vi "dfd_Adjust Height.vi"(9 "origin":cluster{"left":i16, "top":i16}, 10 "fraction rect":T1) -> (2 "rect out":T1)   [LabVIEW 2017, in "NI_DigFilter_Process.lvlib"]
uses:
  <vilib>/addons/Digital Filter Design/NI_DigFilter_Process.lvlib
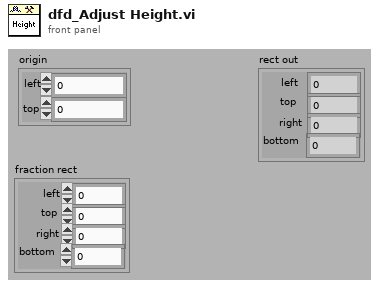
[diagram p1: front panel]
types:
  T1 = cluster{"left":i16, "top":i16, "right":i16, "bottom":i16}
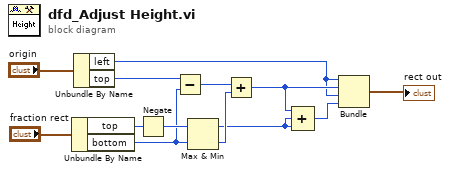
[diagram p0: block diagram]
diagram:
  n1 = Unbundle By Name("fraction rect") -> ("top"=w12:i16, "bottom"=w8:i16)
  n2 = Unbundle By Name("origin") -> ("left"=w3:i16, "top"=w9:i16)
  n3 = Negate(x=w12) -> (-x=w11:i16)
  n4 = Subtract(x=w9, y=w8) -> (x-y=w7:i16)
  n5 = Max & Min(x=w11, y=w8) -> (max(x,y)=w5:i16, min(x,y)=w6:i16)
  n6 = Add(x=w7, y=w6) -> (x+y=w4:i16)
  n7 = Compound Arithmetic op=ADD(w4, w5, w5) -> (w2:i16)
  n8 = Bundle("left"=w3, w4, "left"=w3, w2) -> (→"rect out":cluster{"left":i16, i16, "left":i16, i16})  [unwired: 1 out]
